vi "Write to Hardware.vi"(7 "Valid Triggers":bool, 8 "error in":errorcluster, 9 "Trigger Values":dbl[](array[numeric]), 10 "Values in":dbl[](array[numeric]), 11 "Address Based Execution Unit Implementation in":refnum<class "Address Based Execution Unit.lvclass">) -> (0 "error out":errorcluster, 1 "Trigger Values out":dbl[](array[numeric]), 2 "Values out":dbl[](array[numeric]), 3 "Address Based Execution Unit Implementation out":refnum<class "Address Based Execution Unit.lvclass">)   [LabVIEW 2023, in "Ballard MIL-STD-1553 Engine Support.lvlib" / "Implementation.lvlib" / "Address Based Execution Unit.lvclass"]
uses:
  Address Based Execution Unit.lvclass
  Address Based Execution Unit.lvclass/Address Based Execution Unit.ctl
  Scripting/Constants.vi
  <instrlib>/BTI1553Lib/Private/BC/Data/BC Transmit Acyclic Frame.vi
  <instrlib>/BTI1553Lib/BTI1553LV.lvlib
  Scripting/Ballard MIL-STD-1553 Scripting.lvlib
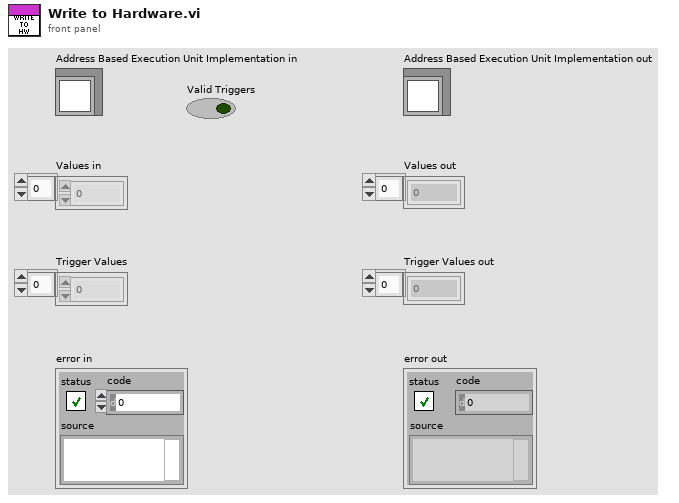
[diagram p1: front panel]
types:
  T1 = typedef "Ballard MIL-STD-1553 Engine Support.lvlib/Implementation.lvlib/Address Based Execution Unit.lvclass/Acyclic Trigger Info.ctl" = cluster{"bus controller handle":u64, "name":string}
  T2 = typedef "Ballard MIL-STD-1553 Engine Support.lvlib/Implementation.lvlib/Address Based Execution Unit.lvclass/Address Write Info.ctl" = cluster{"terminal address":T3, "terminal handle":u64}
  T3 = typedef "Address.ctl" = u16
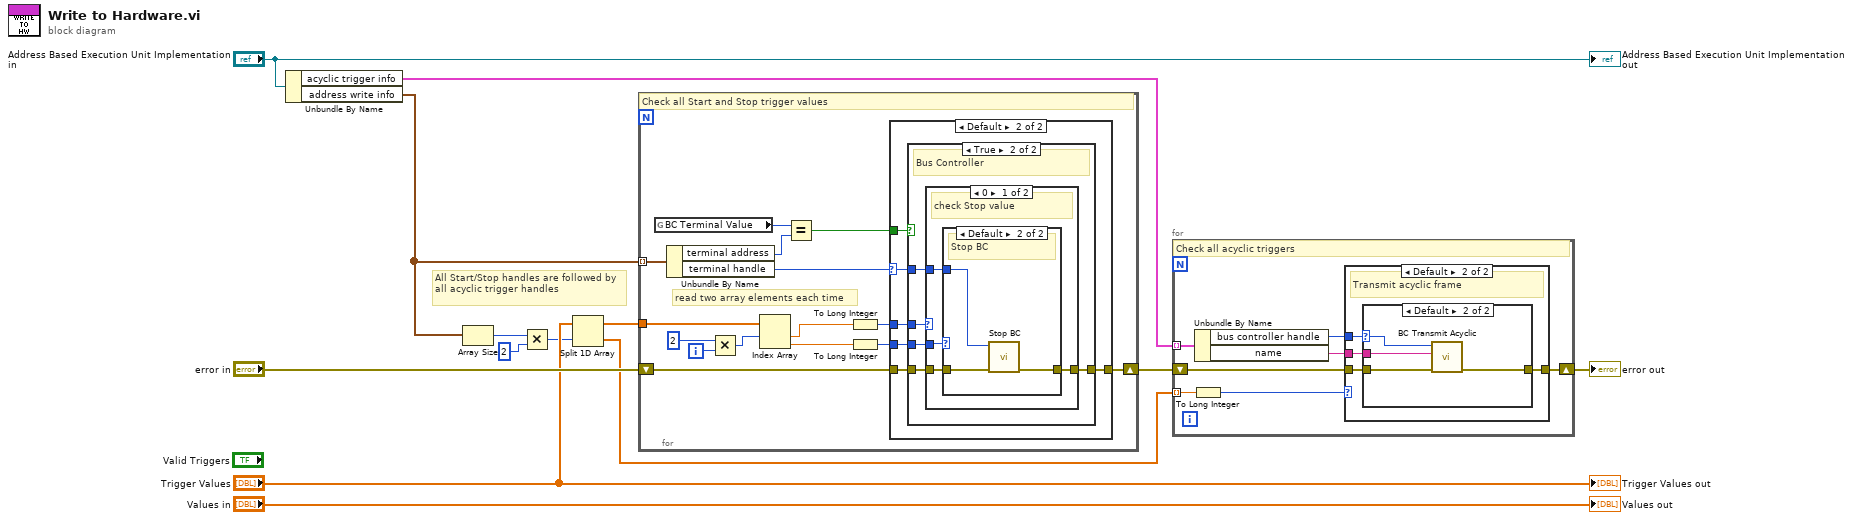
[diagram p0: block diagram]
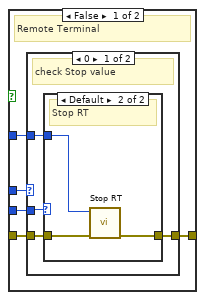
[diagram p5: hidden frame]
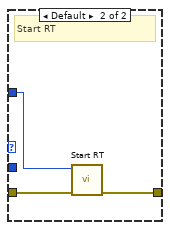
[diagram p7: hidden frame]
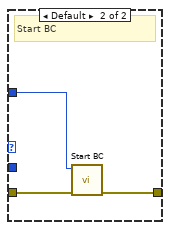
[diagram p9: hidden frame]
diagram:
  # "All Start/Stop handles are followed by all acyclic trigger handles"
  n1 = Unbundle By Name("Address Based Execution Unit Implementation in") -> ("acyclic trigger info"=w1:T1[], "address write info"=w9:T2[])
  n2 = Array Size(array=w9) -> (size(s)=w8:i32)
  n3 = Multiply(x=w8, y=2) -> (x*y=w6:i32)
  n4 = Split 1D Array(array="Trigger Values", index=w6) -> (first subarray=w10:dbl[], second subarray=w2:dbl[])
  n5 = for {
    tunnel: w9 -> [w28] mode=indexing
    shift-right: [w24] -> w5
    shift-left: "error in" -> [w25]
    tunnel: w10 -> [w27]
    i -> [w20]
    # "read two array elements each time"
    # "Check all Start and Stop trigger values"
    n6 = global read "Constants.vi" "BC Terminal Value"() -> (w16:u16)
    n7 = Unbundle By Name(w28) -> ("terminal address"=w15:T3, "terminal handle"=w26:u64)
    n8 = Multiply(x=2, y=w20) -> (x*y=w19:i32)
    n9 = Index Array(array=w27, index #1=w19) -> (element #1=w22:dbl, element #2=w23:dbl)  [unwired: 1 in]
    n10 = Equal?(x=w16, y=w15) -> (x = y?=w14:bool)
    n11 = To Long Integer(number=w22) -> (32bit integer=w18:i32)
    n12 = To Long Integer(number=w23) -> (32bit integer=w17:i32)
    n13 = case shown="Default" w26 {
      selector: w26 -> [_ w35]
      tunnel: w25 -> [w29 w34]
      tunnel: [w29 w33] -> w24
      tunnel: w18 -> [_ w32]
      tunnel: w17 -> [_ w31]
      tunnel: w14 -> [_ w30]
      frame 0, -1 {
      }
      frame Default {
        n14 = case shown="True" w30 {
          tunnel: w32 -> [w40 w56]
          tunnel: w31 -> [w36 w52]
          tunnel: w35 -> [w39 w55]
          tunnel: w34 -> [w38 w54]
          tunnel: [w37 w53] -> w33
          frame False {
            # "Remote Terminal"
            n15 = case shown="0" w40 {
              tunnel: w39 -> [w42 w50]
              tunnel: w38 -> [w43 w51]
              tunnel: [w41 w49] -> w37
              tunnel: w36 -> [w44 _]
              frame 0 {
                # "check Stop value"
                n16 = case shown="Default" w44 {
                  tunnel: w43 -> [w45 w48]
                  tunnel: w42 -> [_ w47]
                  tunnel: [w45 w46] -> w41
                  frame 0 {
                    # "do nothing"
                  }
                  frame Default {
                    # "Stop RT"
                    n17 = call <instrlib>:"Stop RT.vi"("error in (no error)"=w48, "remote terminal handle in"=w47) -> ("error out"=w46:errorcluster)  [unwired: 8 in, 1 out]
                  }
                }
              }
              frame Default {
                # "Start RT"
                n18 = call <instrlib>:"Start RT.vi"("error in (no error)"=w51, "remote terminal handle in"=w50) -> ("error out"=w49:errorcluster)  [unwired: 8 in, 1 out]
              }
            }
          }
          frame True {
            # "Bus Controller"
            n19 = case shown="0" w56 {
              tunnel: w55 -> [w58 w65]
              tunnel: w54 -> [w59 w67]
              tunnel: [w57 w66] -> w53
              tunnel: w52 -> [w60 _]
              frame 0 {
                # "check Stop value"
                n20 = case shown="Default" w60 {
                  tunnel: w59 -> [w61 w64]
                  tunnel: w58 -> [_ w62]
                  tunnel: [w61 w63] -> w57
                  frame 0 {
                    # "do nothing"
                  }
                  frame Default {
                    # "Stop BC"
                    n21 = call <instrlib>:"Stop BC.vi"("error in (no error)"=w64, "bus controller handle in"=w62) -> ("error out"=w63:errorcluster)  [unwired: 8 in, 1 out]
                  }
                }
              }
              frame Default {
                # "Start BC"
                n22 = call <instrlib>:"Start BC.vi"("error in (no error)"=w67, "bus controller handle in"=w65) -> ("error out"=w66:errorcluster)  [unwired: 8 in, 1 out]
              }
            }
          }
        }
      }
    }
  }
  n23 = for {
    shift-right: [w73] -> w4
    shift-left: w5 -> [w74]
    tunnel: w1 -> [w70] mode=indexing
    tunnel: w2 -> [w72] mode=indexing
    # "Check all acyclic triggers"
    n24 = To Long Integer(number=w72) -> (32bit integer=w71:i32)
    n25 = Unbundle By Name(w70) -> ("bus controller handle"=w69:u64, "name"=w68:string)
    n26 = case shown="Default" w71 {
      tunnel: w74 -> [w75 w78]
      tunnel: [w75 w79] -> w73
      tunnel: w69 -> [_ w77]
      tunnel: w68 -> [_ w76]
      frame 0 {
        # "Do nothing"
      }
      frame Default {
        # "Transmit acyclic frame"
        n27 = case shown="Default" w77 {
          selector: w77 -> [_ w83]
          tunnel: [w80 w84] -> w79
          tunnel: w76 -> [_ w82]
          tunnel: w78 -> [w80 w81]
          frame 0, -1 {
          }
          frame Default {
            n28 = call-poly <instrlib>:"BC Transmit Acyclic.vi"("error in (no error)"=w81, "acyclic frame name"=w82, "bus controller handle in"=w83) -> ("error out"=w84:errorcluster)  [unwired: 7 in, 1 out]
          }
        }
      }
    }
  }
  "error out" <- w4
  "Address Based Execution Unit Implementation out" <- "Address Based Execution Unit Implementation in"
  "Values out" <- "Values in"
  "Trigger Values out" <- "Trigger Values"
